vi "SafeClosePins (SubVI).vi"(0 "Lakeshore VISA Refnum in":refnum<visa-resource-name>, 1 "Settings array in":i32[](array[numeric]), 5 "Lakeshore error in (no error)":errorcluster, 7 "Channel Str":string, 9 "Switchboard VISA resource name in":refnum<visa-resource-name>, 11 "Switchboard error in":errorcluster, 12 "Pin array in":dbl[](array[numeric])) -> (3 "Settings array out":i32[](array[numeric]), 4 "Lakeshore VISA Refnum out 2":refnum<visa-resource-name>, 6 "Lakeshore error out 2":errorcluster, 10 "Switchboard VISA Refnum out":refnum<visa-resource-name>, 15 "Switchboard error out":errorcluster)   [LabVIEW 2017, in "Fridge Software v2.1.lvlib"]
uses:
  Fridge Software v2.1.lvlib
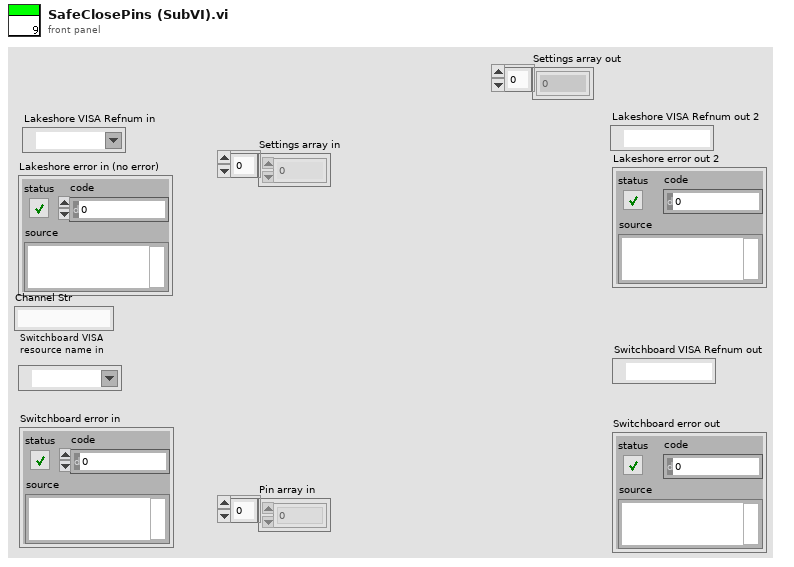
[diagram p1: front panel]
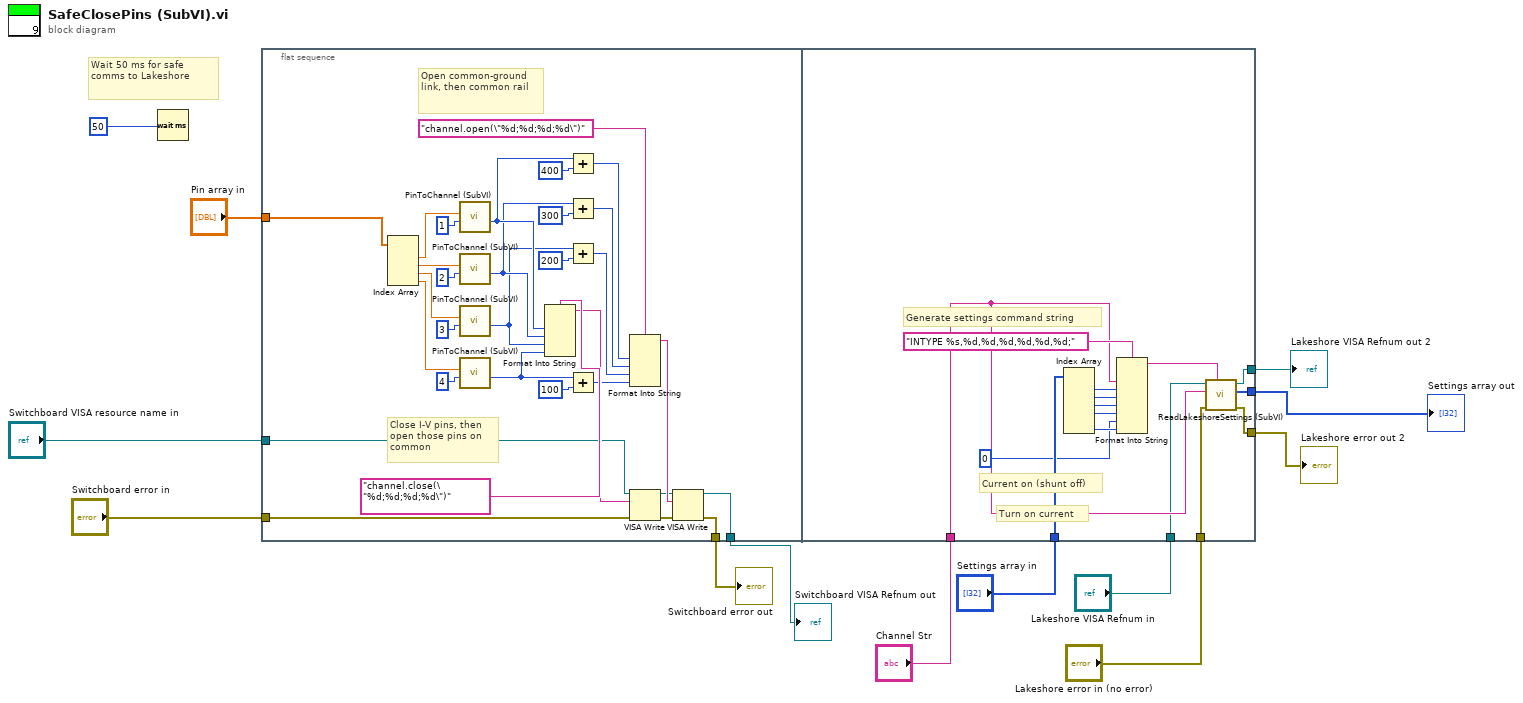
[diagram p0: block diagram]
diagram:
  # "Wait 50 ms for safe comms to Lakeshore"
  n1 = Wait (ms)(milliseconds to wait=50) -> ()  [unwired: 1 out]
  n2 = flat-sequence {
    tunnel: "Switchboard VISA resource name in" -> [w22]
    tunnel: [w21] -> w6
    tunnel: "Switchboard error in" -> [w20]
    tunnel: [w19] -> w8
    tunnel: "Pin array in" -> [w14]
    tunnel: "Channel Str" -> [w51]
    tunnel: "Settings array in" -> [w55]
    tunnel: "Lakeshore VISA Refnum in" -> [w50]
    tunnel: "Lakeshore error in (no error)" -> [w49]
    tunnel: [w47] -> w4
    tunnel: [w46] -> w3
    tunnel: [w45] -> w2
    frame #0 {
      # "Close I-V pins, then open those pins on common"
      # "Open common-ground link, then common rail"
      n3 = Index Array(array=w14) -> (element #1=w18:dbl, element #2=w17:dbl, element #3=w16:dbl, element #4=w15:dbl)  [unwired: 4 in]
      n4 = call "PinToChannel (SubVI).vi"("Pin"=w18, "Slot"=1) -> ("Channel"=w29:i32)  [unwired: 8 in]
      n5 = call "PinToChannel (SubVI).vi"("Pin"=w17, "Slot"=2) -> ("Channel"=w27:i32)  [unwired: 8 in]
      n6 = call "PinToChannel (SubVI).vi"("Pin"=w16, "Slot"=3) -> ("Channel"=w25:i32)  [unwired: 8 in]
      n7 = call "PinToChannel (SubVI).vi"("Pin"=w15, "Slot"=4) -> ("Channel"=w23:i32)  [unwired: 8 in]
      n8 = Format Into String(format string="channel.close(\"%d;%d;%d;%d\")", w29, w27, w25, w23) -> (resulting string=w43:string)  [unwired: 2 in, 1 out]
      n9 = Add(x=w29, y=400) -> (x+y=w34:i32)
      n10 = Add(x=w27, y=300) -> (x+y=w33:i32)
      n11 = Add(x=w25, y=200) -> (x+y=w32:i32)
      n12 = Add(x=w23, y=100) -> (x+y=w31:i32)
      n13 = Format Into String(format string="channel.open(\"%d;%d;%d;%d\")", w34, w33, w32, w31) -> (resulting string=w41:string)  [unwired: 2 in, 1 out]
      n14 = VISA Write(VISA resource name=w22, write buffer=w43, error in (no error)=w20) -> (VISA resource name out=w40:refnum<visa-resource-name>, error out=w39:errorcluster)  [unwired: 1 out]
      n15 = VISA Write(VISA resource name=w40, write buffer=w41, error in (no error)=w39) -> (VISA resource name out=w21:refnum<visa-resource-name>, error out=w19:errorcluster)  [unwired: 1 out]
    }
    frame #1 {
      # "Current on (shunt off)"
      # "Turn on current"
      # "Generate settings command string"
      n16 = Index Array(array=w55) -> (element #1=w59:i32, element #2=w54:i32, element #3=w58:i32, element #4=w57:i32, element #6=w56:i32)  [unwired: 6 in, 1 out]
      n17 = Format Into String(format string="INTYPE %s,%d,%d,%d,%d,%d,%d;", w51, w59, w54, w58, w57, 0, w56) -> (resulting string=w48:string)  [unwired: 2 in, 1 out]
      n18 = call "ReadLakeshoreSettings (SubVI).vi"("Prepended command"=w48, "error in (no error)"=w49, "Channel Str"=w51, "Lakeshore port"=w50) -> ("error out"=w46:errorcluster, "Settings array out"=w45:i32[], "VISA Refnum out"=w47:refnum<visa-resource-name>)  [unwired: 3 in]
    }
  }
  "Switchboard error out" <- w8
  "Switchboard VISA Refnum out" <- w6
  "Lakeshore VISA Refnum out 2" <- w4
  "Lakeshore error out 2" <- w3
  "Settings array out" <- w2
